vi "Open Log File.vi"(8 "error in (no error)":errorcluster, 10 "Path":path, 11 "Log Producer in":refnum<class "Log Producer.lvclass">) -> (0 "error out":errorcluster, 3 "Log Producer out":refnum<class "Log Producer.lvclass">)   [LabVIEW 2020, in "Ballard ARINC 429 Engine.lvlib" / "Implementation.lvlib" / "Word Logging.lvlib" / "Log Producer.lvclass"]
uses:
  Log Producer.lvclass
  Log Producer.lvclass/Log Producer.ctl
  Logger Interface/Logger Interface.lvclass
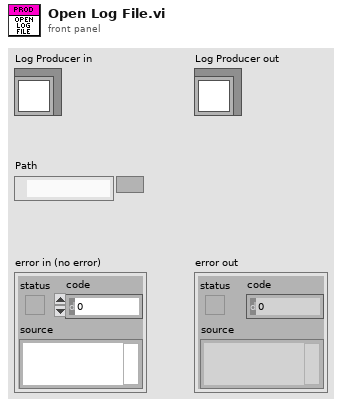
[diagram p1: front panel]
types:
  T1 = typedef "Ballard ARINC 429 Engine.lvlib/Implementation.lvlib/Word Logging.lvlib/Logger Data Reference.ctl" = refnum<data-value>
  T2 = cluster{"Logger Interface":refnum<class "Logger Interface.lvclass">}
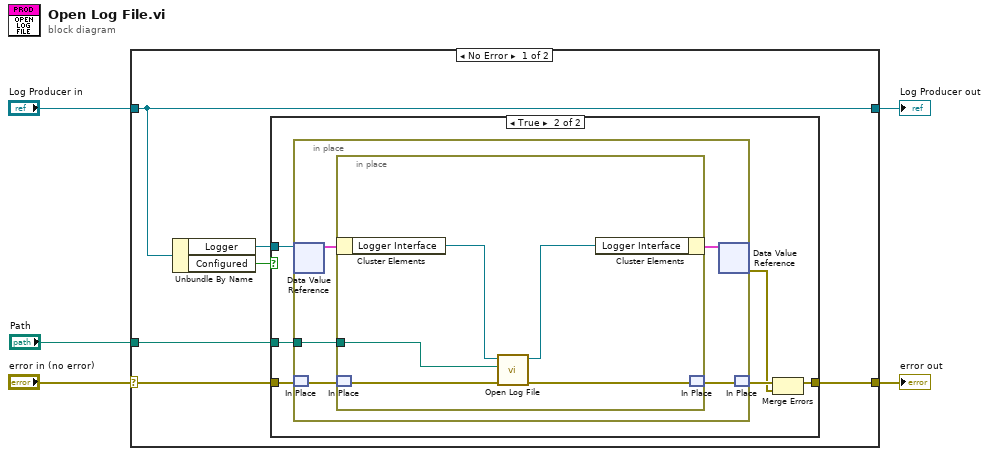
[diagram p0: block diagram]
diagram:
  n1 = case shown="No Error" "error in (no error)" {
    selector: "error in (no error)" -> [w11 w30]
    tunnel: [w8 w30] -> w4
    tunnel: [w10 w29] -> w2
    tunnel: "Log Producer in" -> [w10 w29]
    tunnel: "Path" -> [w7 _]
    frame No Error {
      n2 = Unbundle By Name(w10) -> ("Logger"=w9:T1, "Configured"=w6:bool)
      n3 = case shown="True" w6 {
        tunnel: w11 -> [w12 w18]
        tunnel: w9 -> [_ w17]
        tunnel: [w12 w15] -> w8
        tunnel: w7 -> [_ w13]
        frame False {
        }
        frame True {
          n4 = in-place {
            in-place-border: w13 -> [w19]
            n5 = in-place-dvr #1(w17) -> (w21:T2)  [unwired: 1 out]
            n6 = in-place-match #2(w18) -> (w23:errorcluster)
            n7 = in-place {
              in-place-border: w19 -> [w24]
              n8 = in-place-cluster #3(w21) -> ("Logger Interface"=w26:refnum<class "Logger Interface.lvclass">)
              n9 = in-place-match #4(w23) -> (w28:errorcluster)
              n10 = call-dynamic "Open Log File.vi"("error in (no error)"=w28, "Path"=w24, "Logger Interface in"=w26) -> ("error out"=w27:errorcluster, "Logger Interface out"=w25:refnum<class "Logger Interface.lvclass">)  [unwired: 7 in]
              n11 = in-place-cluster #3("Logger Interface"=w25) -> (w20:T2)
              n12 = in-place-match #4(w27) -> (w22:errorcluster)
            }
            n13 = in-place-dvr #1(w20) -> (w14:errorcluster)  [unwired: 1 out]
            n14 = in-place-match #2(w22) -> (w16:errorcluster)
          }
          n15 = Merge Errors(w16, w14) -> (w15:errorcluster)
        }
      }
    }
    frame Error {
    }
  }
  "error out" <- w4
  "Log Producer out" <- w2
